vi "Resize (ARGB).vi"(7 "Interpolation Mode (Default: CUBIC)":T2=enum."CUBIC", 8 "error in (no error)":errorcluster, 9 "New Image Size":T3, 10 "ARGB Destination Image in":T1, 11 "ARGB Source Image in":T1) -> (0 "error out":errorcluster, 3 "ARGB  Destination Image":T1)   [LabVIEW 2020, in "image.lvlib"]
doc: "Resize the Source Image. The Destination Image will be sized to fit the specified \"New Image Size\"."
uses:
  image.lvlib
  ARGB Image.ctl
  common/Image Size (Integer).ctl
  Interpolation Mode.ctl
  c2d955e4-7b08-44cd-801f-dcd0ae61a3f9.vi
  <vilib>/Utility/error.llb/Error Cluster From Error Code.vi
  common/common.lvlib
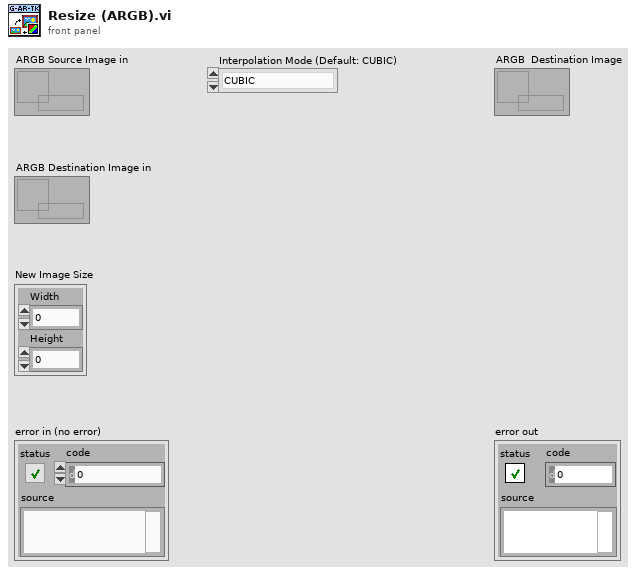
[diagram p1: front panel]
types:
  T1 = typedef "image.lvlib/ARGB Image.ctl" = refnum<data-value>
  T2 = typedef "image.lvlib/Interpolation Mode.ctl" = enum8{"NEAREST", "LINEAR", "CUBIC", "AREA", "LANCZOS", "LINEAR_EXACT", "NEAREST_EXACT", "MAX"}
  T3 = typedef "common.lvlib/Image Size (Integer).ctl" = cluster{"Width":u16, "Height":u16}
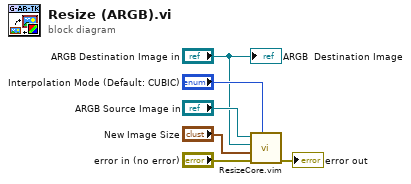
[diagram p0: block diagram]
diagram:
  n1 = call "ResizeCore.vim"("OpenCV Interpolation Flag"="Interpolation Mode (Default: CUBIC)", "error in (no error)"="error in (no error)", "ImageSize"="New Image Size", "Destination Image"="ARGB Destination Image in", "Source Image"="ARGB Source Image in") -> ("error out"=→"error out":errorcluster)  [unwired: 6 in]
  "ARGB  Destination Image" <- "ARGB Destination Image in"
